vi "CRYCalc Rub Buzz THD.vi"(4 "Total Noise":dbl[](array[numeric]), 6 "HT Option":bool[](array[boolean]), 7 "Method":u16, 8 "Amplitude sweep (F)":bool, 9 "Fs":dbl format="%.2f", 10 "Harmonics":dbl[](array[numeric]) format="%.2f", 11 "Freq resp curves":cluster{cluster{"x":dbl, "y":dbl, "z":dbl}[]}[](array[cluster]) {"?"."z" format="%.2f"; "?"."y" format="%#.7g"; "?"."x" format="%.2f"}) -> (0 "Harmonic Track Out":T1(array[cluster]) {"Harmonic Track Data"."?"."z" format="%.2f"; "Harmonic Track Data"."?"."y" format="%.6f"; "Harmonic Track Data"."?"."x" format="%.2f"}, 2 "THD(%)":cluster{cluster{"x":dbl, "y":dbl, "z":dbl}[]}[](array[cluster]) {"?"."z" format="%.2f"; "?"."y" format="%.2f"; "?"."x" format="%.2f"}, 3 "Rub & buzz(%)":cluster{cluster{"x":dbl, "y":dbl, "z":dbl}[]}[](array[cluster]) {"?"."z" format="%.2f"; "?"."y" format="%.2f"; "?"."x" format="%.2f"})   [LabVIEW 2013]
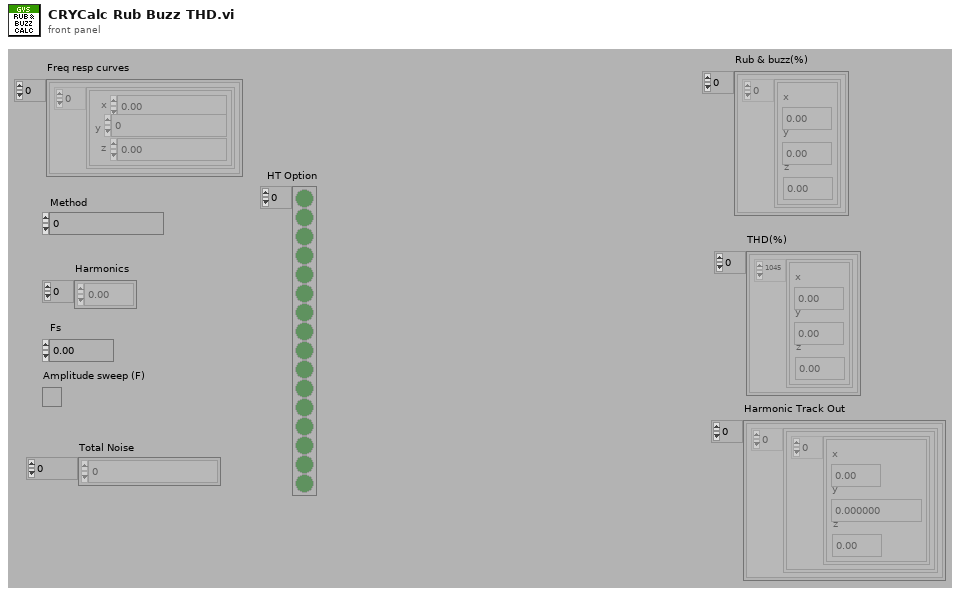
[diagram p1: front panel]
types:
  T1 = cluster{"Harmonic Track Data":cluster{cluster{"x":dbl, "y":dbl, "z":dbl}[]}[]}[]
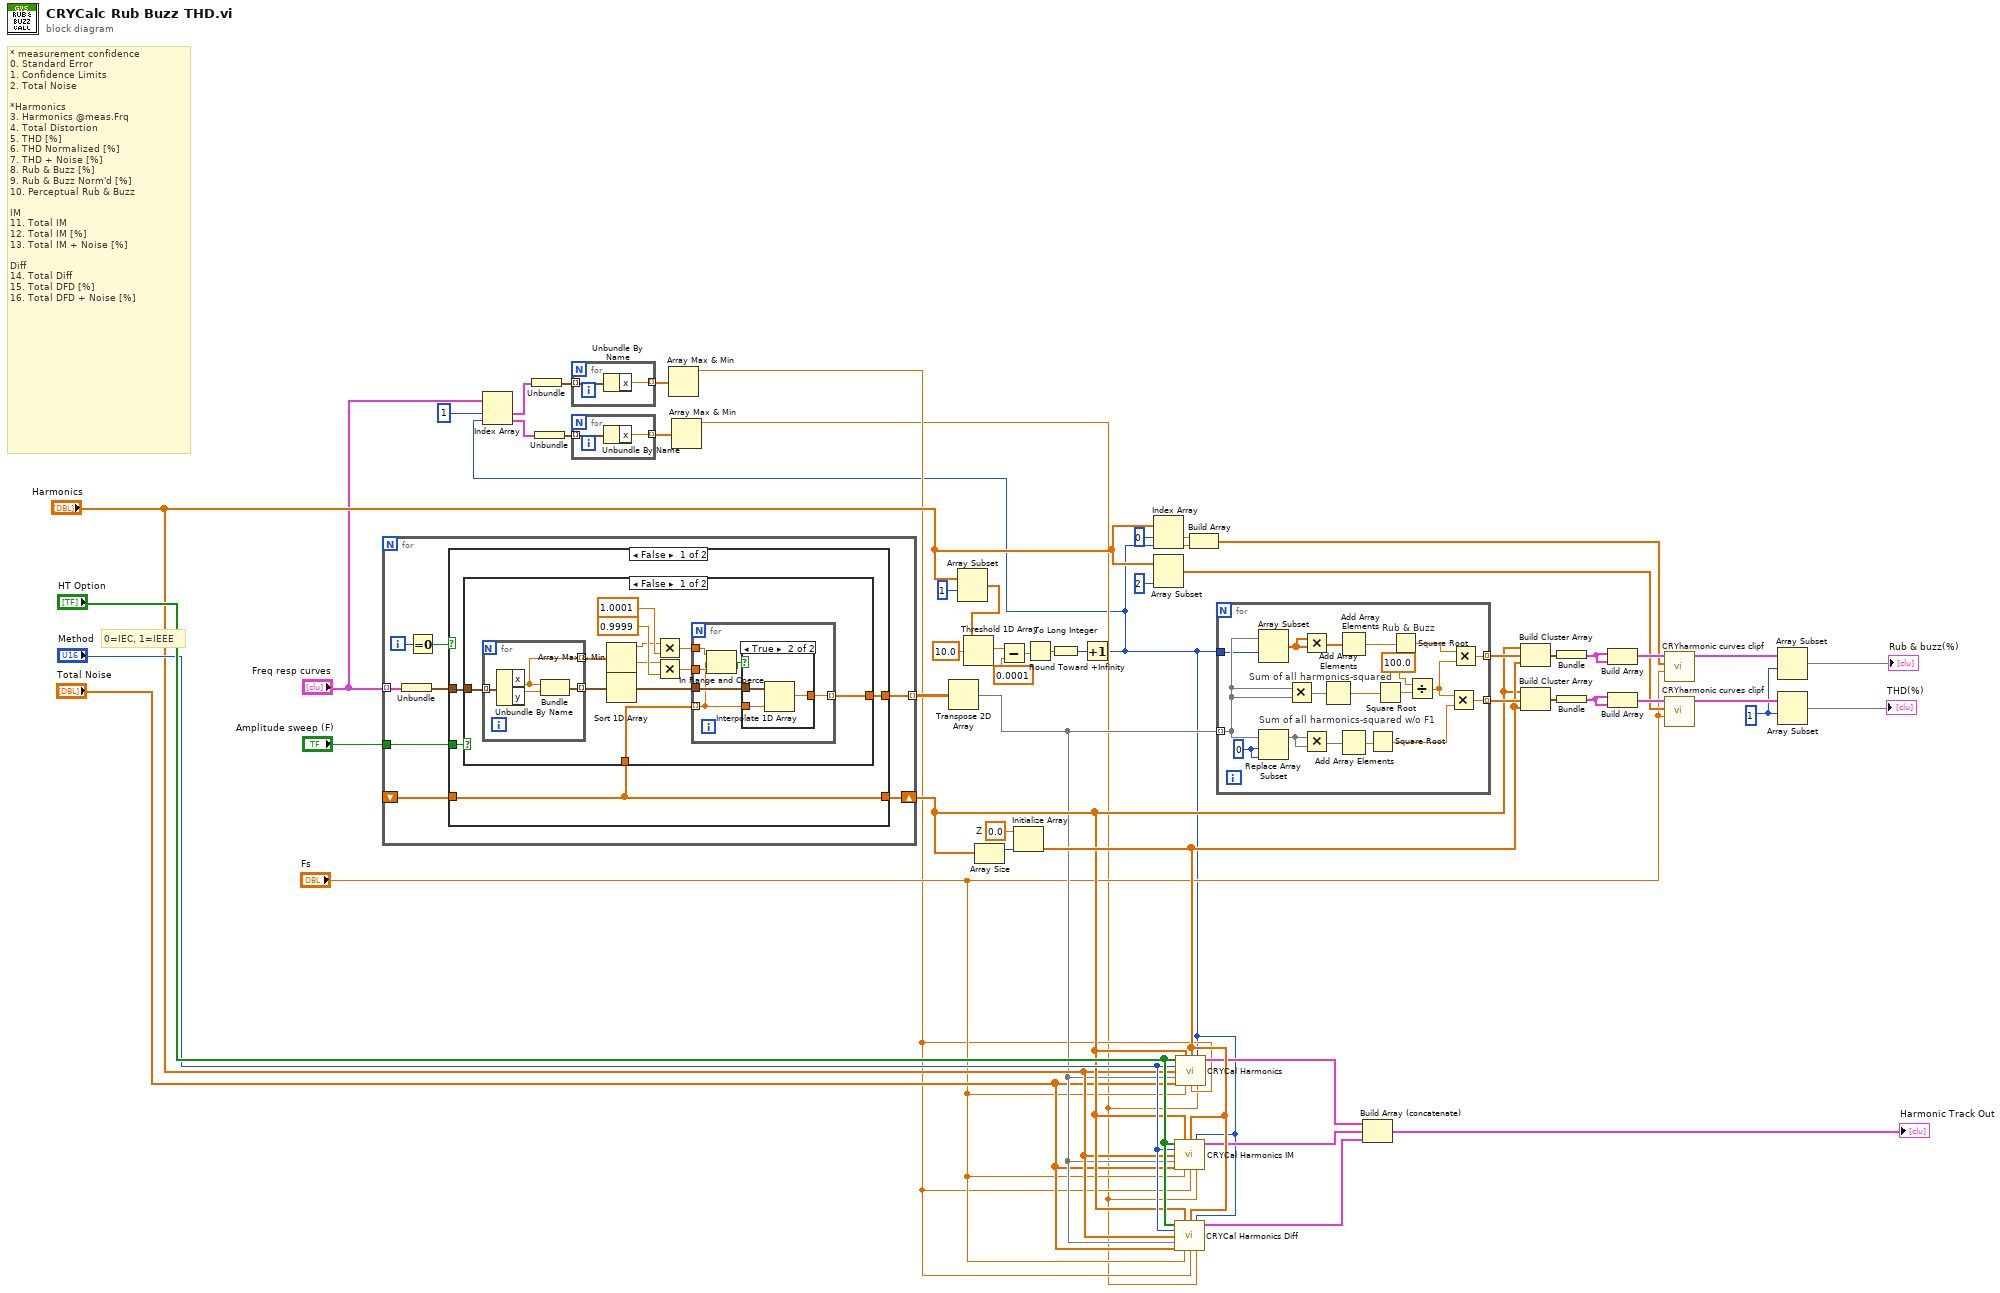
[diagram p0: block diagram]
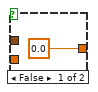
[diagram p2: hidden frame]
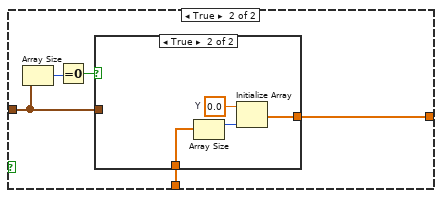
[diagram p3: hidden frame]
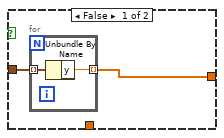
[diagram p4: hidden frame]
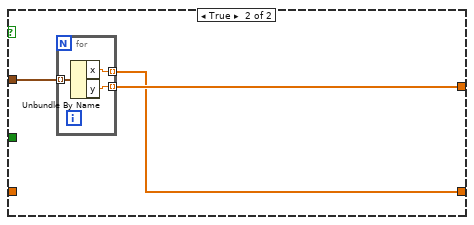
[diagram p5: hidden frame]
diagram:
  w41 = 1 ("Array Index")
  w52 = 0.0  # Z
  # "* measurement confidence\n0. Standard Error\n1. Confidence Limits\n2. Total Noise\n\n*Harmonics\n3. Harmonics @meas.Frq\n4. Total Distortion\n5. THD [%]\n6. THD Normalized [%]\n7. THD + Noise [%]\n8. Rub & Buzz [%]\n9. Rub & Buzz Norm'd [%]\n10. Perceptual Rub & Buzz\n\nIM\n11. Total IM\n12. Total IM [%]\n13. Total IM + Noise [%]\n\nDiff\n14. Total Diff\n15. Total DFD [%]\n16. Total DFD + Noise [%]"
  # "0=IEC, 1=IEEE"
  n1 = for {
    tunnel: "Freq resp curves" -> [w56] mode=indexing
    shift-right: [w61] -> w14
    shift-left: _ -> [w60]
    tunnel: [w58] -> w19 mode=indexing
    tunnel: "Amplitude sweep (F)" -> [w57]
    i -> [w59]
    n2 = Unbundle(w56) -> (w55:cluster{"x":dbl, "y":dbl, "z":dbl}[])
    n3 = Equal To 0?(x=w59) -> (x = 0?=w62:bool)
    n4 = case shown="False" w62 {
      tunnel: w55 -> [w66 w108]
      tunnel: [w64 w106] -> w61
      tunnel: w60 -> [w64 _]
      tunnel: [w65 w107] -> w58
      tunnel: w57 -> [w63 _]
      frame False {
        n5 = case shown="False" w63 {
          tunnel: w66 -> [w78 w97]
          tunnel: [w76 w93] -> w65
          tunnel: w64 -> [w75 w94]
          frame False {
            n6 = for {
              tunnel: w78 -> [w92] mode=indexing
              tunnel: [w90] -> w77 mode=indexing
              tunnel: [w89] -> w74 mode=indexing
              n7 = Unbundle By Name(w92) -> ("x"=w89:dbl, "y"=w91:dbl)
              n8 = Bundle("x"=w89, "y"=w91) -> (w90:cluster{"x":dbl, "y":dbl})  [unwired: 1 out]
            }
            n9 = Array Max & Min(array=w74) -> (max value=w70:dbl, min value=w71:dbl)  [unwired: 2 out]
            n10 = Sort 1D Array(array=w77) -> (sorted array=w67:cluster{"x":dbl, "y":dbl}[])
            n11 = Multiply(x=w70, y=1.0001) -> (x*y=w68:dbl)
            n12 = Multiply(x=w71, y=0.9999) -> (x*y=w69:dbl)
            n13 = for {
              tunnel: w67 -> [w84]
              tunnel: w75 -> [w80] mode=indexing
              tunnel: [w83] -> w76 mode=indexing
              tunnel: w69 -> [w82]
              tunnel: w68 -> [w81]
              n14 = In Range and Coerce(upper limit=w81, x=w80, lower limit=w82) -> (In Range?=w79:bool)  [unwired: 1 out]
              n15 = case shown="True" w79 {
                tunnel: w84 -> [_ w88]
                tunnel: [0.0 w87] -> w83
                tunnel: w80 -> [_ w86]
                frame False {
                }
                frame True {
                  n16 = Interpolate 1D Array(1:w86, 2:w88) -> (0:w87:dbl)
                }
              }
            }
          }
          frame True {
            n17 = Array Size(array=w97) -> (size(s)=w96:i32)
            n18 = Equal To 0?(x=w96) -> (x = 0?=w95:bool)
            n19 = case shown="True" w95 {
              tunnel: w97 -> [w99 _]
              tunnel: w94 -> [_ w103]
              tunnel: [w98 w102] -> w93
              frame False {
                n20 = for {
                  tunnel: w99 -> [w101] mode=indexing
                  tunnel: [w100] -> w98 mode=indexing
                  n21 = Unbundle By Name(w101) -> ("y"=w100:dbl)
                }
              }
              frame True {
                w104 = 0.0  # Y
                n22 = Array Size(array=w103) -> (size(s)=w105:i32)
                n23 = Initialize Array(w104, w105) -> (w102:dbl[])
              }
            }
          }
        }
      }
      frame True {
        n24 = for {
          tunnel: w108 -> [w111] mode=indexing
          tunnel: [w110] -> w107 mode=indexing
          tunnel: [w109] -> w106 mode=indexing
          n25 = Unbundle By Name(w111) -> ("x"=w109:dbl, "y"=w110:dbl)
        }
      }
    }
  }
  n26 = Transpose 2D Array(2D array=w19) -> (transposed array=w12:dbl[][])
  n27 = Array Subset(array="Harmonics", index=1 ("Array Index")) -> (w30:dbl[])  [unwired: 1 in]
  n28 = Threshold 1D Array(2:10.0 ("threshold y"), 3:w30) -> (0:w37:dbl)  [unwired: 1 out]
  n29 = Array Size(array=w14) -> (size(s)=w51:i32)
  n30 = Subtract(x=w37, y=0.0001) -> (x-y=w35:dbl)
  n31 = Initialize Array(w52, w51) -> (w15:dbl[])
  n32 = Round Toward +Infinity(x=w35) -> (ceil(x): smallest int >= x=w53:dbl)
  n33 = To Long Integer(number=w53) -> (32bit integer=w34:i32)
  n34 = Increment(x=w34) -> (x+1=w3:i32)
  n35 = Index Array(array="Freq resp curves", index #1=1 ("index"), index #2=w3) -> (element #1=w26:cluster{cluster{"x":dbl, "y":dbl, "z":dbl}[]}, element #2=w2:cluster{cluster{"x":dbl, "y":dbl, "z":dbl}[]})
  n36 = Unbundle(w26) -> (w25:cluster{"x":dbl, "y":dbl, "z":dbl}[])
  n37 = Unbundle(w2) -> (w22:cluster{"x":dbl, "y":dbl, "z":dbl}[])
  n38 = for {
    tunnel: w25 -> [w113] mode=indexing
    tunnel: [w112] -> w24 mode=indexing
    n39 = Unbundle By Name(w113) -> ("x"=w112:dbl)
  }
  n40 = for {
    tunnel: w22 -> [w115] mode=indexing
    tunnel: [w114] -> w23 mode=indexing
    n41 = Unbundle By Name(w115) -> ("x"=w114:dbl)
  }
  n42 = Array Max & Min(array=w24) -> (max value=w6:dbl)  [unwired: 3 out]
  n43 = Array Max & Min(array=w23) -> (max value=w5:dbl)  [unwired: 3 out]
  n44 = Index Array(array="Harmonics", index #1=0 ("Index"), index #2=w3) -> (element #1=w32:dbl, element #2=w28:dbl)
  n45 = Array Subset(array="Harmonics", length=2 ("Array Length")) -> (w18:dbl[])  [unwired: 1 in]
  n46 = call "CRYCal Harmonics IM.vi"("HT Option"="HT Option", "x"=w14, "z"=w15, "Index"=w3, "Method"="Method", "Harmonic"="Harmonics", "Freq resp curves"=w12, "Total Noise"="Total Noise", "Fs"="Fs", "max value1"=w6, "max value2"=w5) -> ("Harmonic Track Out"=w8:cluster{cluster{cluster[]}[]}[])  [unwired: 4 in]
  n47 = call "CRYCal Harmonics Diff.vi"("HT Option"="HT Option", "x"=w14, "z"=w15, "Index"=w3, "Method"="Method", "Harmonic"="Harmonics", "Freq resp curves"=w12, "Total Noise"="Total Noise", "Fs"="Fs", "max value1"=w6, "max value2"=w5) -> ("Harmonic Track Out"=w7:cluster{cluster{cluster[]}[]}[])  [unwired: 4 in]
  n48 = call "CRYCal Harmonics.vi"("HT Option"="HT Option", "x"=w14, "z"=w15, "Index"=w3, "Method"="Method", "Harmonic"="Harmonics", "Freq resp curves"=w12, "Total Noise"="Total Noise", "Fs"="Fs", "max value1"=w6, "max value2"=w5) -> ("Harmonic Track Out"=w9:cluster{cluster{cluster[]}[]}[])  [unwired: 4 in]
  n49 = Build Array(w32, w28) -> (w29:dbl[])
  n50 = for {
    tunnel: w12 -> [w120] mode=indexing
    tunnel: w3 -> [w119]
    tunnel: [w118] -> w49 mode=indexing
    tunnel: [w117] -> w50 mode=indexing
    w116 = 0
    # "Sum of all harmonics-squared"
    # "Rub & Buzz"
    # "Sum of all harmonics-squared w/o F1"
    n51 = Array Subset(array=w120, index=w119) -> (w126:dbl[])  [unwired: 1 in]
    n52 = Replace Array Subset(array=w120, new element=w116, index=w116) -> (w131:dbl[])
    n53 = Multiply(x=w120, y=w120) -> (x*y=w123:dbl[])
    n54 = Multiply(x=w126, y=w126) -> (x*y=w128:dbl[])
    n55 = Multiply(x=w131, y=w131) -> (x*y=w129:dbl[])
    n56 = Add Array Elements(numeric array=w123) -> (sum=w122:dbl)
    n57 = Add Array Elements(numeric array=w128) -> (sum=w127:dbl)
    n58 = Add Array Elements(numeric array=w129) -> (sum=w130:dbl)
    n59 = Square Root(x=w130) -> (sqrt(x)=w133:dbl)
    n60 = Square Root(x=w122) -> (sqrt(x)=w121:dbl)
    n61 = Square Root(x=w127) -> (sqrt(x)=w124:dbl)
    n62 = Divide(x=100.0, y=w121) -> (x/y=w125:dbl)
    n63 = Multiply(x=w125, y=w133) -> (x*y=w117:dbl)
    n64 = Multiply(x=w124, y=w125) -> (x*y=w118:dbl)
  }
  n65 = Build Array (concatenate)(w9, w8, w7) -> (→"Harmonic Track Out":cluster{cluster{cluster[]}[]}[])
  n66 = Build Cluster Array(w14, w49, w15) -> (w48:cluster{"x":dbl, dbl, "Z":dbl}[])
  n67 = Build Cluster Array(w14, w50, w15) -> (w47:cluster{"x":dbl, dbl, "Z":dbl}[])
  n68 = Bundle(w48) -> (w40:cluster{cluster{"x":dbl, dbl, "Z":dbl}[]})  [unwired: 1 in]
  n69 = Bundle(w47) -> (w46:cluster{cluster{"x":dbl, dbl, "Z":dbl}[]})  [unwired: 1 in]
  n70 = Build Array(w40, w40) -> (w39:cluster{cluster{"x":dbl, dbl, "Z":dbl}[]}[])
  n71 = Build Array(w46, w46) -> (w45:cluster{cluster{"x":dbl, dbl, "Z":dbl}[]}[])
  n72 = call "CRYharmonic curves clipf.vi"("Fs"="Fs", "Harmonics"=w29, "Freq resp curves"=w39) -> ("Freq resp curves clipped"=w42:cluster{cluster{"x":dbl, "y":dbl, "z":dbl}[]}[])  [unwired: 8 out]
  n73 = call "CRYharmonic curves clipf.vi"("Fs"="Fs", "Harmonics"=w18, "Freq resp curves"=w45) -> ("Freq resp curves clipped"=w44:cluster{cluster{"x":dbl, "y":dbl, "z":dbl}[]}[])  [unwired: 8 out]
  n74 = Array Subset(array=w42, index=w41) -> (→"Rub & buzz(%)":cluster{cluster{"x":dbl, "y":dbl, "z":dbl}[]}[])  [unwired: 1 in]
  n75 = Array Subset(array=w44, index=w41) -> (→"THD(%)":cluster{cluster{"x":dbl, "y":dbl, "z":dbl}[]}[])  [unwired: 1 in]
